vi "FeedbackDecode_ParseMSMSXML.vi"(1 "XMLFile":path) -> (0 "ComponentArray":T1(array[cluster])=[{"Name"="", "Type"="", "ID"="", "Num"="", "COM"=[], "Offset"=[], "RotationAxis"=[], "OrientationMatrix"=[], "MinAngle"=0.0, "MaxAngle"=0.0, "InboardID"="", "InboardNum"="", "InboardCOM"=[], "OutboardID"="", "OutboardNum"="", "OutboardCOM"=[]}, {"Name"="\"sphere\"", "Type"="\"Trans3Joint\"", "ID"="J", "Num"="102", "COM"=[], "Offset"=[], "RotationAxis"=[], "OrientationMatrix"=[[1.0, 0.0, 0.0], [0.0, 1.0, 0.0], [0.0, 0.0, 1.0]], "MinAngle"=0.0, "MaxAngle"=0.0, "InboardID"="", "InboardNum"="", "InboardCOM"=[], "OutboardID"="", "OutboardNum"="", "OutboardCOM"=[]}, {"Name"="\"Ulna\"", "Type"="\"Segment\"", "ID"="S", "Num"="10", "COM"=[0.0, -0.05, 0.0], "Offset"=[0.0, -0.125, 0.0], "RotationAxis"=[], "OrientationMatrix"=[], "MinAngle"=0.0, "MaxAngle"=0.0, "InboardID"="", "InboardNum"="", "InboardCOM"=[], "OutboardID"="", "OutboardNum"="", "OutboardCOM"=[]}, {"Name"="\"Humerus\"", "Type"="\"Segment\"", "ID"="S", "Num"="6", "COM"=[0.0, -0.05, 0.0], "Offset"=[0.0, -0.125, 0.0], "RotationAxis"=[], "OrientationMatrix"=[], "MinAngle"=0.0, "MaxAngle"=0.0, "InboardID"="", "InboardNum"="", "InboardCOM"=[], "OutboardID"="", "OutboardNum"="", "OutboardCOM"=[]}, {"Name"="\"Sphere\"", "Type"="\"Segment\"", "ID"="S", "Num"="100", "COM"=[0.0, 0.0, 0.0], "Offset"=[0.0, -0.125, 0.0], "RotationAxis"=[], "OrientationMatrix"=[], "MinAngle"=0.0, "MaxAngle"=0.0, "InboardID"="", "InboardNum"="", "InboardCOM"=[], "OutboardID"="", "OutboardNum"="", "OutboardCOM"=[]}, {"Name"="\"Elbow Flexor\"", "Type"="\"Muscle\"", "ID"="M", "Num"="9", "COM"=[], "Offset"=[], "RotationAxis"=[], "OrientationMatrix"=[], "MinAngle"=0.0, "MaxAngle"=0.0, "InboardID"="", "InboardNum"="", "InboardCOM"=[], "OutboardID"="", "OutboardNum"="", "OutboardCOM"=[]}, {"Name"="\"Shoulder\"", "Type"="\"PinJoint\"", "ID"="J", "Num"="7", "COM"=[], "Offset"=[], "RotationAxis"=[0.0, 0.0, 1.0], "OrientationMatrix"=[[1.0, 0.0, 0.0], [0.0, 1.0, 0.0], [0.0, 0.0, 1.0]], "MinAngle"=0.0, "MaxAngle"=0.0, "InboardID"="", "InboardNum"="", "InboardCOM"=[], "OutboardID"="", "OutboardNum"="", "OutboardCOM"=[]}])   [LabVIEW 2020]
uses:
  <vilib>/regexp/Match Regular Expression.xnode
panel:
  in  "Component":T2
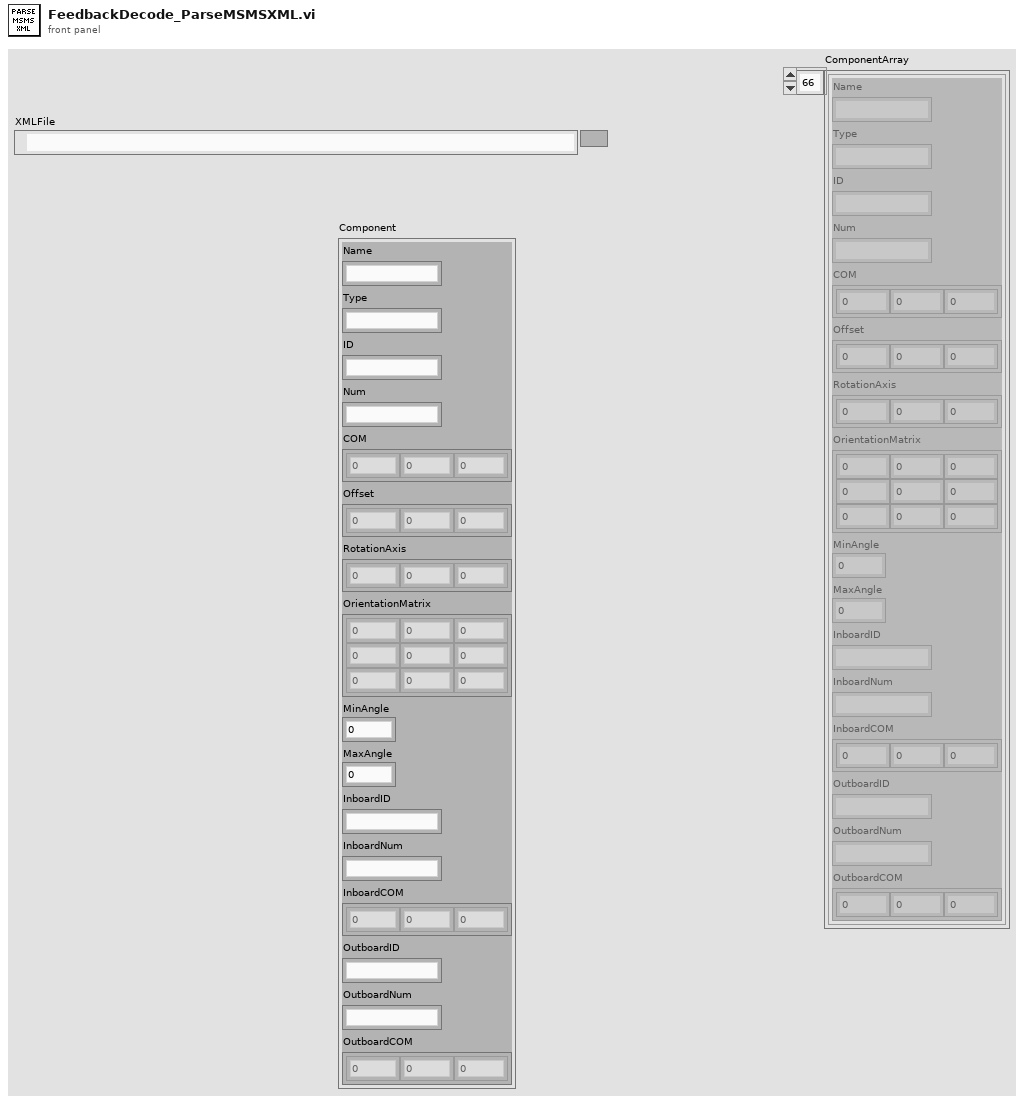
[diagram p1: front panel]
types:
  T1 = cluster{"Name":string, "Type":string, "ID":string, "Num":string, "COM":dbl[], "Offset":dbl[], "RotationAxis":dbl[], "OrientationMatrix":dbl[][], "MinAngle":dbl, "MaxAngle":dbl, "InboardID":string, "InboardNum":string, "InboardCOM":dbl[], "OutboardID":string, "OutboardNum":string, "OutboardCOM":dbl[]}[]
  T2 = cluster{"Name":string, "Type":string, "ID":string, "Num":string, "COM":dbl[], "Offset":dbl[], "RotationAxis":dbl[], "OrientationMatrix":dbl[][], "MinAngle":dbl, "MaxAngle":dbl, "InboardID":string, "InboardNum":string, "InboardCOM":dbl[], "OutboardID":string, "OutboardNum":string, "OutboardCOM":dbl[]}
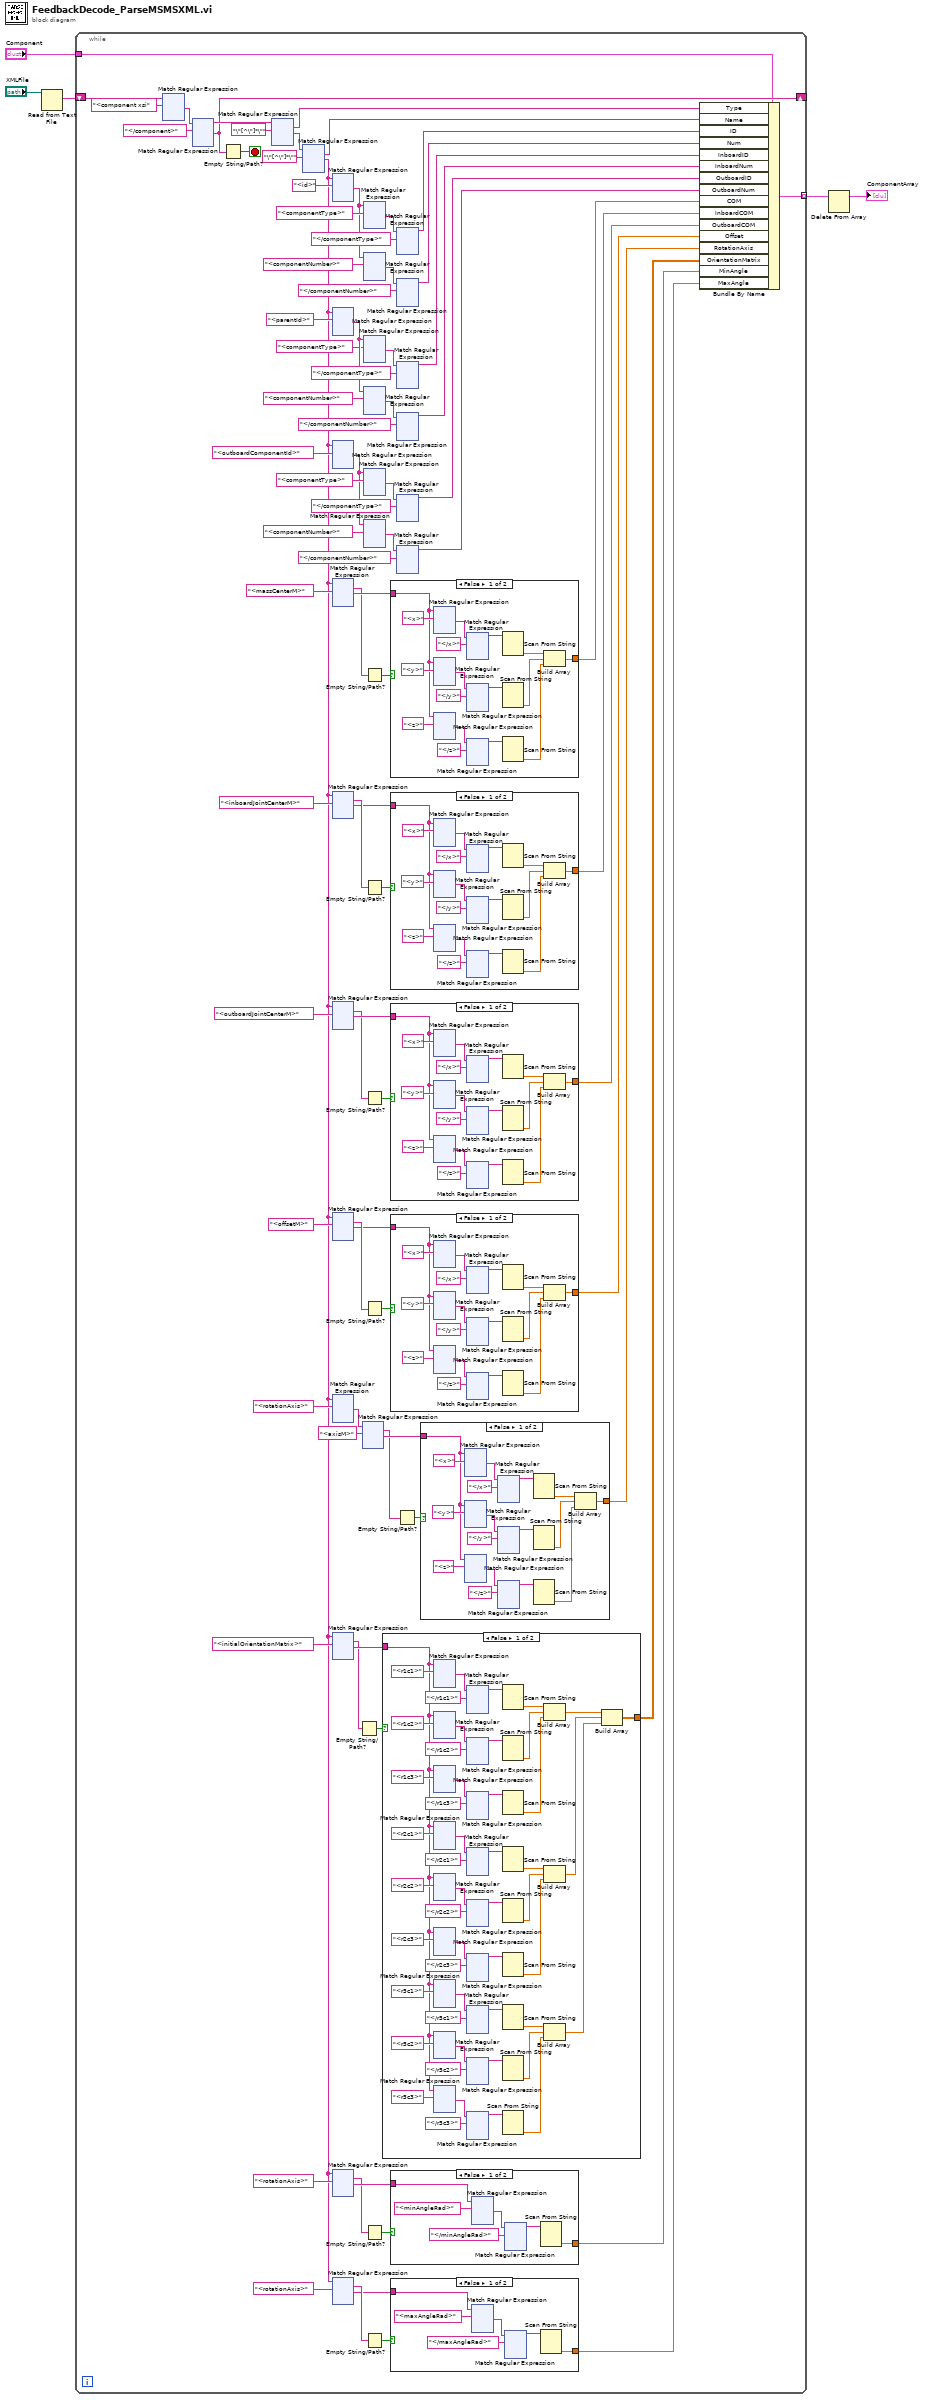
[diagram p0: block diagram]
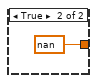
[diagram p2: hidden frame]
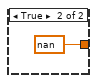
[diagram p3: hidden frame]
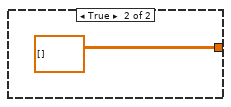
[diagram p4: hidden frame]
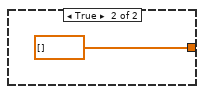
[diagram p5: hidden frame]
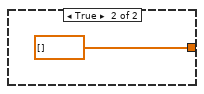
[diagram p6: hidden frame]
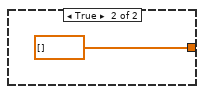
[diagram p7: hidden frame]
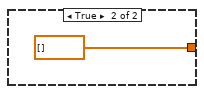
[diagram p8: hidden frame]
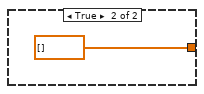
[diagram p9: hidden frame]
diagram:
  n1 = Read from Text File(file (use dialog)="XMLFile") -> (text=w4:string)  [unwired: 3 in, 3 out]
  n2 = while {
    shift-right: [w86] -> _
    shift-left: w4 -> [w92]
    tunnel: "Component" -> [w83]
    tunnel: [w82] -> w2 mode=indexing
    stop <- w85 stop-if-true
    n3 = xnode "Match Regular Expression"("input string"=w92, "regular expression"="<component xsi") -> ("after match"=w90:string)  [unwired: 4 in, 4 out]
    n4 = xnode "Match Regular Expression"("input string"=w90, "regular expression"="</component>") -> ("before match"=w87:string, "after match"=w86:string)  [unwired: 4 in, 3 out]
    n5 = Empty String/Path?(string/path=w86) -> (empty?=w85:bool)
    n6 = xnode "Match Regular Expression"("input string"=w87, "regular expression"="\"[^\"]*\"") -> ("whole match"=w81:string, "after match"=w79:string)  [unwired: 4 in, 3 out]
    n7 = xnode "Match Regular Expression"("input string"=w79, "regular expression"="\"[^\"]*\"") -> ("whole match"=w80:string, "after match"=w6:string)  [unwired: 4 in, 3 out]
    n8 = xnode "Match Regular Expression"("input string"=w6, "regular expression"="<id>") -> ("after match"=w70:string)  [unwired: 4 in, 4 out]
    n9 = xnode "Match Regular Expression"("input string"=w6, "regular expression"="<parentId>") -> ("after match"=w68:string)  [unwired: 4 in, 4 out]
    n10 = xnode "Match Regular Expression"("input string"=w6, "regular expression"="<outboardComponentId>") -> ("after match"=w51:string)  [unwired: 4 in, 4 out]
    n11 = xnode "Match Regular Expression"("input string"=w6, "regular expression"="<massCenterM>") -> ("whole match"=w44:string, "after match"=w47:string)  [unwired: 4 in, 3 out]
    n12 = xnode "Match Regular Expression"("input string"=w6, "regular expression"="<inboardJointCenterM>") -> ("whole match"=w43:string, "after match"=w41:string)  [unwired: 4 in, 3 out]
    n13 = xnode "Match Regular Expression"("input string"=w6, "regular expression"="<outboardJointCenterM>") -> ("whole match"=w36:string, "after match"=w38:string)  [unwired: 4 in, 3 out]
    n14 = xnode "Match Regular Expression"("input string"=w6, "regular expression"="<offsetM>") -> ("whole match"=w33:string, "after match"=w31:string)  [unwired: 4 in, 3 out]
    n15 = xnode "Match Regular Expression"("input string"=w6, "regular expression"="<rotationAxis>") -> ("after match"=w26:string)  [unwired: 4 in, 4 out]
    n16 = xnode "Match Regular Expression"("input string"=w6, "regular expression"="<initialOrientationMatrix>") -> ("whole match"=w18:string, "after match"=w20:string)  [unwired: 4 in, 3 out]
    n17 = xnode "Match Regular Expression"("input string"=w6, "regular expression"="<rotationAxis>") -> ("whole match"=w13:string, "after match"=w15:string)  [unwired: 4 in, 3 out]
    n18 = xnode "Match Regular Expression"("input string"=w6, "regular expression"="<rotationAxis>") -> ("whole match"=w12:string, "after match"=w10:string)  [unwired: 4 in, 3 out]
    n19 = Empty String/Path?(string/path=w18) -> (empty?=w19:bool)
    n20 = xnode "Match Regular Expression"("input string"=w26, "regular expression"="<axisM>") -> ("whole match"=w23:string, "after match"=w24:string)  [unwired: 4 in, 3 out]
    n21 = xnode "Match Regular Expression"("input string"=w70, "regular expression"="<componentType>") -> ("after match"=w75:string)  [unwired: 4 in, 4 out]
    n22 = xnode "Match Regular Expression"("input string"=w70, "regular expression"="<componentNumber>") -> ("after match"=w73:string)  [unwired: 4 in, 4 out]
    n23 = xnode "Match Regular Expression"("input string"=w68, "regular expression"="<componentType>") -> ("after match"=w64:string)  [unwired: 4 in, 4 out]
    n24 = xnode "Match Regular Expression"("input string"=w68, "regular expression"="<componentNumber>") -> ("after match"=w65:string)  [unwired: 4 in, 4 out]
    n25 = xnode "Match Regular Expression"("input string"=w51, "regular expression"="<componentType>") -> ("after match"=w55:string)  [unwired: 4 in, 4 out]
    n26 = xnode "Match Regular Expression"("input string"=w51, "regular expression"="<componentNumber>") -> ("after match"=w54:string)  [unwired: 4 in, 4 out]
    n27 = Empty String/Path?(string/path=w44) -> (empty?=w45:bool)
    n28 = Empty String/Path?(string/path=w43) -> (empty?=w42:bool)
    n29 = Empty String/Path?(string/path=w36) -> (empty?=w37:bool)
    n30 = Empty String/Path?(string/path=w33) -> (empty?=w32:bool)
    n31 = Empty String/Path?(string/path=w13) -> (empty?=w14:bool)
    n32 = Empty String/Path?(string/path=w12) -> (empty?=w11:bool)
    n33 = case shown="False" w19 {
      tunnel: w20 -> [w795 _]
      tunnel: [w791 dbl[][] []] -> w17
      frame False {
        n34 = xnode "Match Regular Expression"("input string"=w795, "regular expression"="<r1c1>") -> ("after match"=w837:string)  [unwired: 4 in, 4 out]
        n35 = xnode "Match Regular Expression"("input string"=w795, "regular expression"="<r1c2>") -> ("after match"=w838:string)  [unwired: 4 in, 4 out]
        n36 = xnode "Match Regular Expression"("input string"=w795, "regular expression"="<r1c3>") -> ("after match"=w834:string)  [unwired: 4 in, 4 out]
        n37 = xnode "Match Regular Expression"("input string"=w795, "regular expression"="<r2c1>") -> ("after match"=w814:string)  [unwired: 4 in, 4 out]
        n38 = xnode "Match Regular Expression"("input string"=w795, "regular expression"="<r2c2>") -> ("after match"=w813:string)  [unwired: 4 in, 4 out]
        n39 = xnode "Match Regular Expression"("input string"=w795, "regular expression"="<r2c3>") -> ("after match"=w817:string)  [unwired: 4 in, 4 out]
        n40 = xnode "Match Regular Expression"("input string"=w795, "regular expression"="<r3c1>") -> ("after match"=w807:string)  [unwired: 4 in, 4 out]
        n41 = xnode "Match Regular Expression"("input string"=w795, "regular expression"="<r3c2>") -> ("after match"=w808:string)  [unwired: 4 in, 4 out]
        n42 = xnode "Match Regular Expression"("input string"=w795, "regular expression"="<r3c3>") -> ("after match"=w804:string)  [unwired: 4 in, 4 out]
        n43 = xnode "Match Regular Expression"("input string"=w837, "regular expression"="</r1c1>") -> ("before match"=w831:string)  [unwired: 4 in, 4 out]
        n44 = xnode "Match Regular Expression"("input string"=w838, "regular expression"="</r1c2>") -> ("before match"=w830:string)  [unwired: 4 in, 4 out]
        n45 = xnode "Match Regular Expression"("input string"=w834, "regular expression"="</r1c3>") -> ("before match"=w829:string)  [unwired: 4 in, 4 out]
        n46 = xnode "Match Regular Expression"("input string"=w814, "regular expression"="</r2c1>") -> ("before match"=w820:string)  [unwired: 4 in, 4 out]
        n47 = xnode "Match Regular Expression"("input string"=w813, "regular expression"="</r2c2>") -> ("before match"=w821:string)  [unwired: 4 in, 4 out]
        n48 = xnode "Match Regular Expression"("input string"=w817, "regular expression"="</r2c3>") -> ("before match"=w822:string)  [unwired: 4 in, 4 out]
        n49 = xnode "Match Regular Expression"("input string"=w807, "regular expression"="</r3c1>") -> ("before match"=w801:string)  [unwired: 4 in, 4 out]
        n50 = xnode "Match Regular Expression"("input string"=w808, "regular expression"="</r3c2>") -> ("before match"=w800:string)  [unwired: 4 in, 4 out]
        n51 = xnode "Match Regular Expression"("input string"=w804, "regular expression"="</r3c3>") -> ("before match"=w799:string)  [unwired: 4 in, 4 out]
        n52 = Scan From String(input string=w831) -> (output 1=w828:dbl)  [unwired: 4 in, 3 out]
        n53 = Scan From String(input string=w830) -> (output 1=w827:dbl)  [unwired: 4 in, 3 out]
        n54 = Scan From String(input string=w829) -> (output 1=w826:dbl)  [unwired: 4 in, 3 out]
        n55 = Scan From String(input string=w820) -> (output 1=w823:dbl)  [unwired: 4 in, 3 out]
        n56 = Scan From String(input string=w821) -> (output 1=w824:dbl)  [unwired: 4 in, 3 out]
        n57 = Scan From String(input string=w822) -> (output 1=w825:dbl)  [unwired: 4 in, 3 out]
        n58 = Scan From String(input string=w801) -> (output 1=w798:dbl)  [unwired: 4 in, 3 out]
        n59 = Scan From String(input string=w800) -> (output 1=w797:dbl)  [unwired: 4 in, 3 out]
        n60 = Scan From String(input string=w799) -> (output 1=w796:dbl)  [unwired: 4 in, 3 out]
        n61 = Build Array(w828, w827, w826) -> (w794:dbl[])
        n62 = Build Array(w823, w824, w825) -> (w793:dbl[])
        n63 = Build Array(w798, w797, w796) -> (w792:dbl[])
        n64 = Build Array(w794, w793, w792) -> (w791:dbl[][])
      }
      frame True {
      }
    }
    n65 = case shown="False" w45 {
      tunnel: w47 -> [w6393 _]
      tunnel: [w6386 dbl[] []] -> w46
      frame False {
        n66 = xnode "Match Regular Expression"("input string"=w6393, "regular expression"="<x>") -> ("after match"=w6399:string)  [unwired: 4 in, 4 out]
        n67 = xnode "Match Regular Expression"("input string"=w6393, "regular expression"="<y>") -> ("after match"=w6400:string)  [unwired: 4 in, 4 out]
        n68 = xnode "Match Regular Expression"("input string"=w6393, "regular expression"="<z>") -> ("after match"=w6396:string)  [unwired: 4 in, 4 out]
        n69 = xnode "Match Regular Expression"("input string"=w6399, "regular expression"="</x>") -> ("before match"=w6392:string)  [unwired: 4 in, 4 out]
        n70 = xnode "Match Regular Expression"("input string"=w6400, "regular expression"="</y>") -> ("before match"=w6391:string)  [unwired: 4 in, 4 out]
        n71 = xnode "Match Regular Expression"("input string"=w6396, "regular expression"="</z>") -> ("before match"=w6390:string)  [unwired: 4 in, 4 out]
        n72 = Scan From String(input string=w6392) -> (output 1=w6389:dbl)  [unwired: 4 in, 3 out]
        n73 = Scan From String(input string=w6391) -> (output 1=w6388:dbl)  [unwired: 4 in, 3 out]
        n74 = Scan From String(input string=w6390) -> (output 1=w6387:dbl)  [unwired: 4 in, 3 out]
        n75 = Build Array(w6389, w6388, w6387) -> (w6386:dbl[])
      }
      frame True {
      }
    }
    n76 = case shown="False" w42 {
      tunnel: w41 -> [w5577 _]
      tunnel: [w5570 dbl[] []] -> w35
      frame False {
        n77 = xnode "Match Regular Expression"("input string"=w5577, "regular expression"="<x>") -> ("after match"=w5583:string)  [unwired: 4 in, 4 out]
        n78 = xnode "Match Regular Expression"("input string"=w5577, "regular expression"="<y>") -> ("after match"=w5584:string)  [unwired: 4 in, 4 out]
        n79 = xnode "Match Regular Expression"("input string"=w5577, "regular expression"="<z>") -> ("after match"=w5580:string)  [unwired: 4 in, 4 out]
        n80 = xnode "Match Regular Expression"("input string"=w5583, "regular expression"="</x>") -> ("before match"=w5576:string)  [unwired: 4 in, 4 out]
        n81 = xnode "Match Regular Expression"("input string"=w5584, "regular expression"="</y>") -> ("before match"=w5575:string)  [unwired: 4 in, 4 out]
        n82 = xnode "Match Regular Expression"("input string"=w5580, "regular expression"="</z>") -> ("before match"=w5574:string)  [unwired: 4 in, 4 out]
        n83 = Scan From String(input string=w5576) -> (output 1=w5573:dbl)  [unwired: 4 in, 3 out]
        n84 = Scan From String(input string=w5575) -> (output 1=w5572:dbl)  [unwired: 4 in, 3 out]
        n85 = Scan From String(input string=w5574) -> (output 1=w5571:dbl)  [unwired: 4 in, 3 out]
        n86 = Build Array(w5573, w5572, w5571) -> (w5570:dbl[])
      }
      frame True {
      }
    }
    n87 = case shown="False" w37 {
      tunnel: w38 -> [w4761 _]
      tunnel: [w4754 dbl[] []] -> w34
      frame False {
        n88 = xnode "Match Regular Expression"("input string"=w4761, "regular expression"="<x>") -> ("after match"=w4767:string)  [unwired: 4 in, 4 out]
        n89 = xnode "Match Regular Expression"("input string"=w4761, "regular expression"="<y>") -> ("after match"=w4768:string)  [unwired: 4 in, 4 out]
        n90 = xnode "Match Regular Expression"("input string"=w4761, "regular expression"="<z>") -> ("after match"=w4764:string)  [unwired: 4 in, 4 out]
        n91 = xnode "Match Regular Expression"("input string"=w4767, "regular expression"="</x>") -> ("before match"=w4760:string)  [unwired: 4 in, 4 out]
        n92 = xnode "Match Regular Expression"("input string"=w4768, "regular expression"="</y>") -> ("before match"=w4759:string)  [unwired: 4 in, 4 out]
        n93 = xnode "Match Regular Expression"("input string"=w4764, "regular expression"="</z>") -> ("before match"=w4758:string)  [unwired: 4 in, 4 out]
        n94 = Scan From String(input string=w4760) -> (output 1=w4757:dbl)  [unwired: 4 in, 3 out]
        n95 = Scan From String(input string=w4759) -> (output 1=w4756:dbl)  [unwired: 4 in, 3 out]
        n96 = Scan From String(input string=w4758) -> (output 1=w4755:dbl)  [unwired: 4 in, 3 out]
        n97 = Build Array(w4757, w4756, w4755) -> (w4754:dbl[])
      }
      frame True {
      }
    }
    n98 = case shown="False" w32 {
      tunnel: w31 -> [w3945 _]
      tunnel: [w3938 dbl[] []] -> w29
      frame False {
        n99 = xnode "Match Regular Expression"("input string"=w3945, "regular expression"="<x>") -> ("after match"=w3951:string)  [unwired: 4 in, 4 out]
        n100 = xnode "Match Regular Expression"("input string"=w3945, "regular expression"="<y>") -> ("after match"=w3952:string)  [unwired: 4 in, 4 out]
        n101 = xnode "Match Regular Expression"("input string"=w3945, "regular expression"="<z>") -> ("after match"=w3948:string)  [unwired: 4 in, 4 out]
        n102 = xnode "Match Regular Expression"("input string"=w3951, "regular expression"="</x>") -> ("before match"=w3944:string)  [unwired: 4 in, 4 out]
        n103 = xnode "Match Regular Expression"("input string"=w3952, "regular expression"="</y>") -> ("before match"=w3943:string)  [unwired: 4 in, 4 out]
        n104 = xnode "Match Regular Expression"("input string"=w3948, "regular expression"="</z>") -> ("before match"=w3942:string)  [unwired: 4 in, 4 out]
        n105 = Scan From String(input string=w3944) -> (output 1=w3941:dbl)  [unwired: 4 in, 3 out]
        n106 = Scan From String(input string=w3943) -> (output 1=w3940:dbl)  [unwired: 4 in, 3 out]
        n107 = Scan From String(input string=w3942) -> (output 1=w3939:dbl)  [unwired: 4 in, 3 out]
        n108 = Build Array(w3941, w3940, w3939) -> (w3938:dbl[])
      }
      frame True {
      }
    }
    n109 = case shown="False" w14 {
      tunnel: w15 -> [w444 _]
      tunnel: [w442 nan] -> w8
      frame False {
        n110 = xnode "Match Regular Expression"("input string"=w444, "regular expression"="<minAngleRad>") -> ("after match"=w447:string)  [unwired: 4 in, 4 out]
        n111 = xnode "Match Regular Expression"("input string"=w447, "regular expression"="</minAngleRad>") -> ("before match"=w443:string)  [unwired: 4 in, 4 out]
        n112 = Scan From String(input string=w443) -> (output 1=w442:dbl)  [unwired: 4 in, 3 out]
      }
      frame True {
      }
    }
    n113 = case shown="False" w11 {
      tunnel: w10 -> [w95 _]
      tunnel: [w93 nan] -> w7
      frame False {
        n114 = xnode "Match Regular Expression"("input string"=w95, "regular expression"="<maxAngleRad>") -> ("after match"=w98:string)  [unwired: 4 in, 4 out]
        n115 = xnode "Match Regular Expression"("input string"=w98, "regular expression"="</maxAngleRad>") -> ("before match"=w94:string)  [unwired: 4 in, 4 out]
        n116 = Scan From String(input string=w94) -> (output 1=w93:dbl)  [unwired: 4 in, 3 out]
      }
      frame True {
      }
    }
    n117 = Empty String/Path?(string/path=w23) -> (empty?=w27:bool)
    n118 = xnode "Match Regular Expression"("input string"=w75, "regular expression"="</componentType>") -> ("before match"=w74:string)  [unwired: 4 in, 4 out]
    n119 = xnode "Match Regular Expression"("input string"=w73, "regular expression"="</componentNumber>") -> ("before match"=w69:string)  [unwired: 4 in, 4 out]
    n120 = xnode "Match Regular Expression"("input string"=w64, "regular expression"="</componentType>") -> ("before match"=w60:string)  [unwired: 4 in, 4 out]
    n121 = xnode "Match Regular Expression"("input string"=w65, "regular expression"="</componentNumber>") -> ("before match"=w59:string)  [unwired: 4 in, 4 out]
    n122 = xnode "Match Regular Expression"("input string"=w55, "regular expression"="</componentType>") -> ("before match"=w50:string)  [unwired: 4 in, 4 out]
    n123 = xnode "Match Regular Expression"("input string"=w54, "regular expression"="</componentNumber>") -> ("before match"=w49:string)  [unwired: 4 in, 4 out]
    n124 = case shown="False" w27 {
      tunnel: w24 -> [w3129 _]
      tunnel: [w3122 dbl[] []] -> w22
      frame False {
        n125 = xnode "Match Regular Expression"("input string"=w3129, "regular expression"="<x>") -> ("after match"=w3135:string)  [unwired: 4 in, 4 out]
        n126 = xnode "Match Regular Expression"("input string"=w3129, "regular expression"="<y>") -> ("after match"=w3136:string)  [unwired: 4 in, 4 out]
        n127 = xnode "Match Regular Expression"("input string"=w3129, "regular expression"="<z>") -> ("after match"=w3132:string)  [unwired: 4 in, 4 out]
        n128 = xnode "Match Regular Expression"("input string"=w3135, "regular expression"="</x>") -> ("before match"=w3128:string)  [unwired: 4 in, 4 out]
        n129 = xnode "Match Regular Expression"("input string"=w3136, "regular expression"="</y>") -> ("before match"=w3127:string)  [unwired: 4 in, 4 out]
        n130 = xnode "Match Regular Expression"("input string"=w3132, "regular expression"="</z>") -> ("before match"=w3126:string)  [unwired: 4 in, 4 out]
        n131 = Scan From String(input string=w3128) -> (output 1=w3125:dbl)  [unwired: 4 in, 3 out]
        n132 = Scan From String(input string=w3127) -> (output 1=w3124:dbl)  [unwired: 4 in, 3 out]
        n133 = Scan From String(input string=w3126) -> (output 1=w3123:dbl)  [unwired: 4 in, 3 out]
        n134 = Build Array(w3125, w3124, w3123) -> (w3122:dbl[])
      }
      frame True {
      }
    }
    n135 = Bundle By Name(cluster=w83, "Type"=w81, "Name"=w80, "ID"=w74, "Num"=w69, "InboardID"=w60, "InboardNum"=w59, "OutboardID"=w50, "OutboardNum"=w49, "COM"=w46, "InboardCOM"=w35, "OutboardCOM"=w34, "Offset"=w29, "RotationAxis"=w22, "OrientationMatrix"=w17, "MinAngle"=w8, "MaxAngle"=w7) -> (w82:T2)
  }
  n136 = Delete From Array(array=w2) -> (array with subset deleted=→"ComponentArray":T1)  [unwired: 2 in, 1 out]
